vi "flattenedGrid.vi"(0 "z Coordinates":dbl[](array[numeric]), 1 "y Coordinates":dbl[](array[numeric]), 2 "x Layer Number":dbl, 3 "Initial Length x":dbl, 4 "x Delta Length":dbl) -> (5 "Array":dbl[][](array[numeric]))   [LabVIEW 2017]
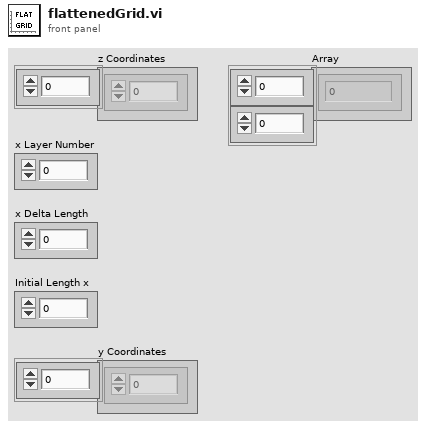
[diagram p1: front panel]
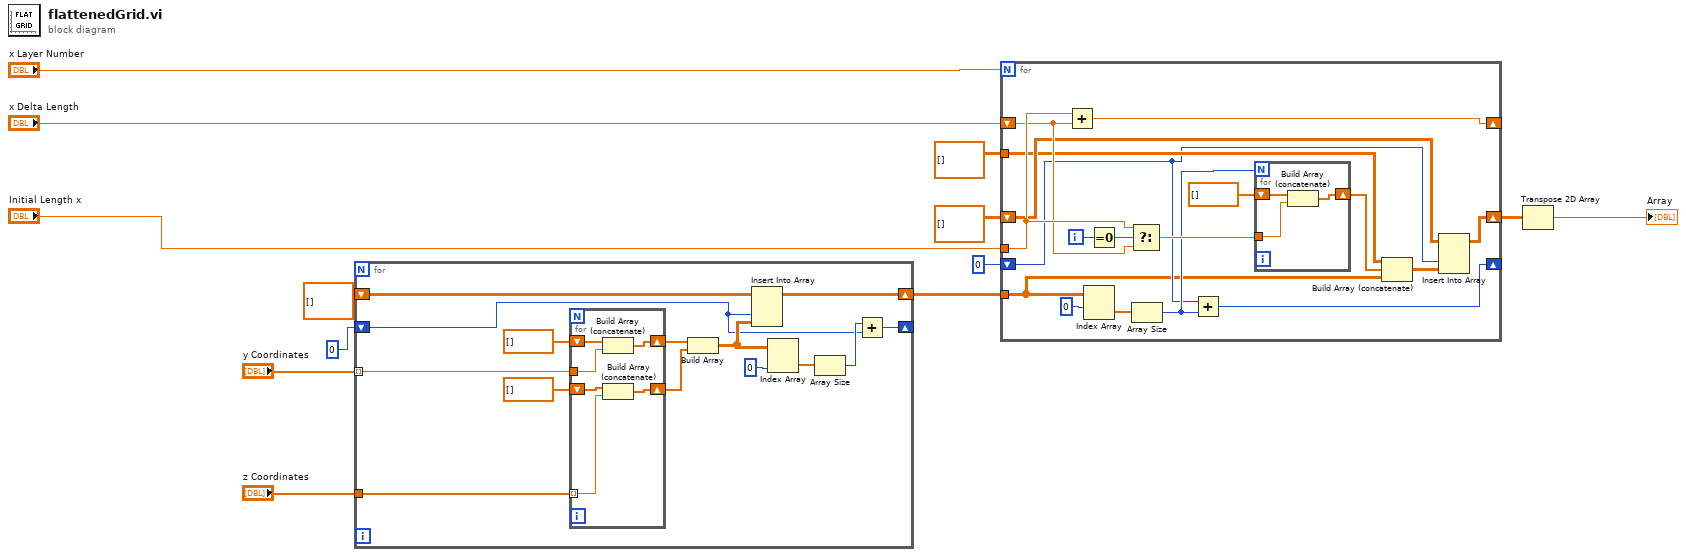
[diagram p0: block diagram]
diagram:
  n1 = for {
    tunnel: "y Coordinates" -> [w26] mode=indexing
    tunnel: "z Coordinates" -> [w27]
    shift-right: [w21] -> w9
    shift-left: dbl[][] [] -> [w20]
    shift-right: [w17] -> _
    shift-left: 0 -> [w14]
    n2 = for {
      tunnel: w27 -> [w29] mode=indexing
      tunnel: w26 -> [w33]
      shift-right: [w32] -> w23
      shift-left: dbl[] [] -> [w31]
      shift-right: [w28] -> w22
      shift-left: dbl[] [] -> [w30]
      n3 = Build Array (concatenate)(w31, w33) -> (w32:dbl[])
      n4 = Build Array (concatenate)(w30, w29) -> (w28:dbl[])
    }
    n5 = Build Array(w23, w22) -> (w16:dbl[][])
    n6 = Insert Into Array(array=w20, index (col)=w14, new element=w16) -> (w21:dbl[][])  [unwired: 1 in]
    n7 = Index Array(array=w16, index (col)=0 ("index (row)")) -> (element=w19:dbl[])  [unwired: 1 in]
    n8 = Array Size(array=w19) -> (size(s)=w18:i32)
    n9 = Add(x=w18, y=w14) -> (x+y=w17:i32)
  }
  n10 = for {
    N: "x Layer Number" -> [_]
    tunnel: w9 -> [w34]
    tunnel: "Initial Length x" -> [w45]
    shift-right: [w48] -> _
    shift-left: "x Delta Length" -> [w44]
    shift-right: [w41] -> w12
    shift-left: dbl[][] [] -> [w42]
    shift-right: [w39] -> _
    shift-left: 0 -> [w36]
    tunnel: dbl[][] [] -> [w38]
    i -> [w46]
    n11 = Add(x=w45, y=w44) -> (x+y=w48:dbl)
    n12 = Index Array(array=w34, index (row)=0) -> (element=w51:dbl[])  [unwired: 1 in]
    n13 = Equal To 0?(x=w46) -> (x = 0?=w47:bool)
    n14 = Select(t=w45, s=w47, f=w44) -> (s? t:f=w43:dbl)
    n15 = Array Size(array=w51) -> (size(s)=w40:i32)
    n16 = Add(x=w36, y=w40) -> (x+y=w39:i32)
    n17 = for {
      N: w40 -> [_]
      tunnel: w43 -> [w54]
      shift-right: [w52] -> w35
      shift-left: dbl[] [] -> [w53]
      n18 = Build Array (concatenate)(w53, w54) -> (w52:dbl[])
    }
    n19 = Build Array (concatenate)(w38, w35, w34) -> (w37:dbl[][])
    n20 = Insert Into Array(array=w42, index (col)=w36, new element=w37) -> (w41:dbl[][])  [unwired: 1 in]
  }
  n21 = Transpose 2D Array(2D array=w12) -> (transposed array=→"Array":dbl[][])
